vi "SCMP - Write FITS File v2 coop.vi"(6 "FITS Header":T1={"Wavelength (nm)"=530.15, "Exposure (s)"=0.05, "Tuning Delay (ms)"=1000.0, "Beam Type (-1/1)"=1.0, "Tuning Voltages"=[1.111, 2.222, 3.333, 4.444], "Observer"="observer", "Light Shapping Diffuser"=enum."In Beam", "Comment"="", "Data Type"=enum."HOLE", "Mod Cycles"=0, "SCD Calibration Optics"=enum."1 - Polarizer @0, I+Q", "SCD Emission Line Filter"=enum."1-557.6nm", "Cookbook"="", "COMP-S Calibration Wheel"=enum."Dark", "COMP-S Andover Filter Wheel"=enum."530.3nm/HWB 0.34nm (Fe XIV)", "FOV Rotation (deg)"=66.0, "Objective Lens Position (mm)"=0.0, "Occulter size"=0.0, "Time End"=timestamp(3382374145.421875 s since 1904-01-01), "Acc Exposure (s)"=0.0, "Time Stamp Array"=[], "Camera Serial Number"=[], "Camera Temp"=[], "Camera PI (mm)"=[], "Time Start"=timestamp(3382374145.421875 s since 1904-01-01), "Peripherals"={"ILX controler"=FALSE, "Zone temperatures"=FALSE, "Andor"=FALSE, "Andor 2"=FALSE, "PI Stages"=FALSE, "AISAS mechanisms"=FALSE, "AISAS Mech.lvclass"=refnum, "Zone temp ref"=variant, "FWs"=FALSE}, "FITS paths"=[], "Cameras"=enum."Andor", "load preset cbk"=FALSE, "periodic check count"=0, "COMP-S Calibration Wheel 2"=enum."Dark", "Calib"=enum."Dark", "Abso Aperture"=66.0, "Nominal Aperture"=66.0} {"Nominal Aperture" format="%.1f"; "Abso Aperture" format="%.1f"; "Camera PI (mm)" format="%_3g"; "Acc Exposure (s)" format="%^.3g"; "Occulter size" format="%.2f"; "Objective Lens Position (mm)" min=70.0 max=152.0 format="%.2f"; "FOV Rotation (deg)" format="%.1f"; "Exposure (s)" format="%^.3g"; "Wavelength (nm)" format="%_6g"}, 8 "error in":errorcluster, 9 "Image #":i32, 10 "Data":u32[][][](array[numeric]), 11 "Camera.lvclass":refnum<class "Camera.lvclass">) -> (0 "error out":errorcluster, 2 "FITS Path Out":path=path "G:/SCD Data/Level-0/20141030/20141030.160747.FTS")   [LabVIEW 2014]
doc: "Use this template to build a VI to use as a subVI."
uses:
  Controls/SCD - FITS Cluster.ctl
  AISAS/Mech/AISAS Mech.lvclass
  AISAS/Controls/Diffuser.ctl
  Controls/FITS Data type.ctl
  Controls/SCD - Calibration Optics Filter Wheel.ctl
  Controls/SCD - EDT - Emission Line Filter Wheel.ctl
  Controls/CoMP-S Controls/Polarization Optics Filter Wheel.ctl
  Controls/CoMP-S Controls/Emission Line Filter Wheel.ctl
  AISAS/Controls/focus.ctl
  Controls/peripherals.ctl
  Controls/Cameras select.ctl
  Camera/Camera/Camera.lvclass
panel:
  out "<ADU>":dbl[](array[numeric])
  in  "A":u32[][](array[numeric])
  in  "D":u32[][](array[numeric])
  in  "C":u32[][](array[numeric])
  in  "B":u32[][](array[numeric])
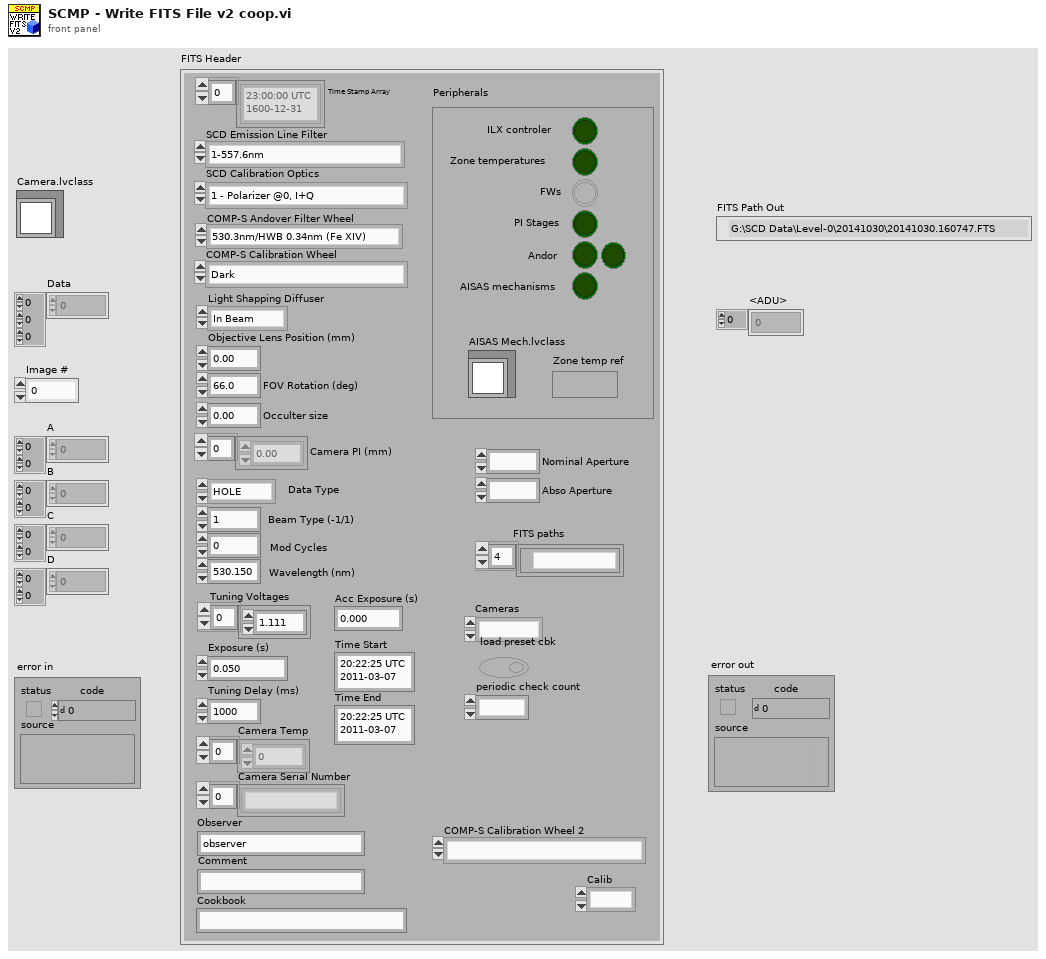
[diagram p1: front panel]
types:
  T1 = typedef "SCD - FITS Cluster.ctl" = cluster{"Wavelength (nm)":dbl, "Exposure (s)":dbl, "Tuning Delay (ms)":dbl, "Beam Type (-1/1)":dbl, "Tuning Voltages":dbl[], "Observer":string, "Light Shapping Diffuser":T2, "Comment":string, "Data Type":T3, "Mod Cycles":u16, "SCD Calibration Optics":T4, "SCD Emission Line Filter":T5, "Cookbook":string, "COMP-S Calibration Wheel":T6, "COMP-S Andover Filter Wheel":T7, "FOV Rotation (deg)":dbl, "Objective Lens Position (mm)":T8, "Occulter size":dbl, "Time End":timestamp, "Acc Exposure (s)":dbl, "Time Stamp Array":timestamp[], "Camera Serial Number":string[], "Camera Temp":dbl[], "Camera PI (mm)":dbl[], "Time Start":timestamp, "Peripherals":T9, "FITS paths":path[], "Cameras":T10, "load preset cbk":bool, "periodic check count":i32, "COMP-S Calibration Wheel 2":T6, "Calib":enum16{"Dark", "Flat"}, "Abso Aperture":dbl, "Nominal Aperture":dbl}
  T2 = typedef "Diffuser.ctl" = enum16{"Out of Beam", "In Beam"}
  T3 = typedef "FITS Data type.ctl" = enum16{"LIVE", "DARK", "FLAT", "CALI", "OBSE", "ABSO", "AURE", "TARG", "OBJE", "HOLE", "OREX", "THRO", "CHIP"}
  T4 = typedef "SCD - Calibration Optics Filter Wheel.ctl" = enum16{"1 - Polarizer @0, I+Q", "2 - Polarizer @90, I-Q", "3 - Polarizer @45, I+U", "4 - Polarizer @135, I-U", "5 - Polarizer @0, Retarder @45, I+V", "6 - Polarizer @0, Retarder @135, I-V", "7 - Dark", "8 - Clear", "9 - N/A"}
  T5 = typedef "SCD - EDT - Emission Line Filter Wheel.ctl" = enum16{"1-557.6nm", "2-587.6nm", "3-589.6nm", "4-630.2nm", "5-656.4nm", "6-849.8nm", "7-854.2nm", "8-866.2nm", "9-1083.0nm"}
  T6 = typedef "Polarization Optics Filter Wheel.ctl" = enum16{"Dark", "Clear", "Exchange Lens", "Polarizer @0, I+Q", "Polarizer @90, I-Q", "Polarizer @45, I+U", "Polarizer @135, I-U", "Polarizer @0, Retarder @45, I+V", "Polarizer @0, Retarder @135, I-V"}
  T7 = typedef "Emission Line Filter Wheel.ctl" = enum16{"530.3nm/HWB 0.34nm (Fe XIV)", "587.6nm/HBW 0.44nm (He I D3)", "637.5nm/HBW 0.53nm (Fe X)", "656.3nm/HBW 0.57nm (H-Alpha)", "789.2nm/HBW 0.85nm (Fe XI)", "854.2nm/HBW 1.01nm (Ca I)", "1074.7nm/HBW 2.34nm (Fe XIII)", "1079.8nm/HBW 1.64nm (Fe XIII)", "1083.0nm/HBW 1.66nm (He I)"}
  T8 = typedef "focus.ctl" = dbl
  T9 = typedef "peripherals.ctl" = cluster{"ILX controler":bool, "Zone temperatures":bool, "Andor":bool, "Andor 2":bool, "PI Stages":bool, "AISAS mechanisms":bool, "AISAS Mech.lvclass":refnum<class "AISAS Mech.lvclass">, "Zone temp ref":variant, "FWs":bool}
  T10 = typedef "Cameras select.ctl" = enum16{"Andor", "GDR"}
  T11 = typedef "beaning.ctl" = enum16{"1x1", "2x2", "3x3", "4x4", "8x8"}
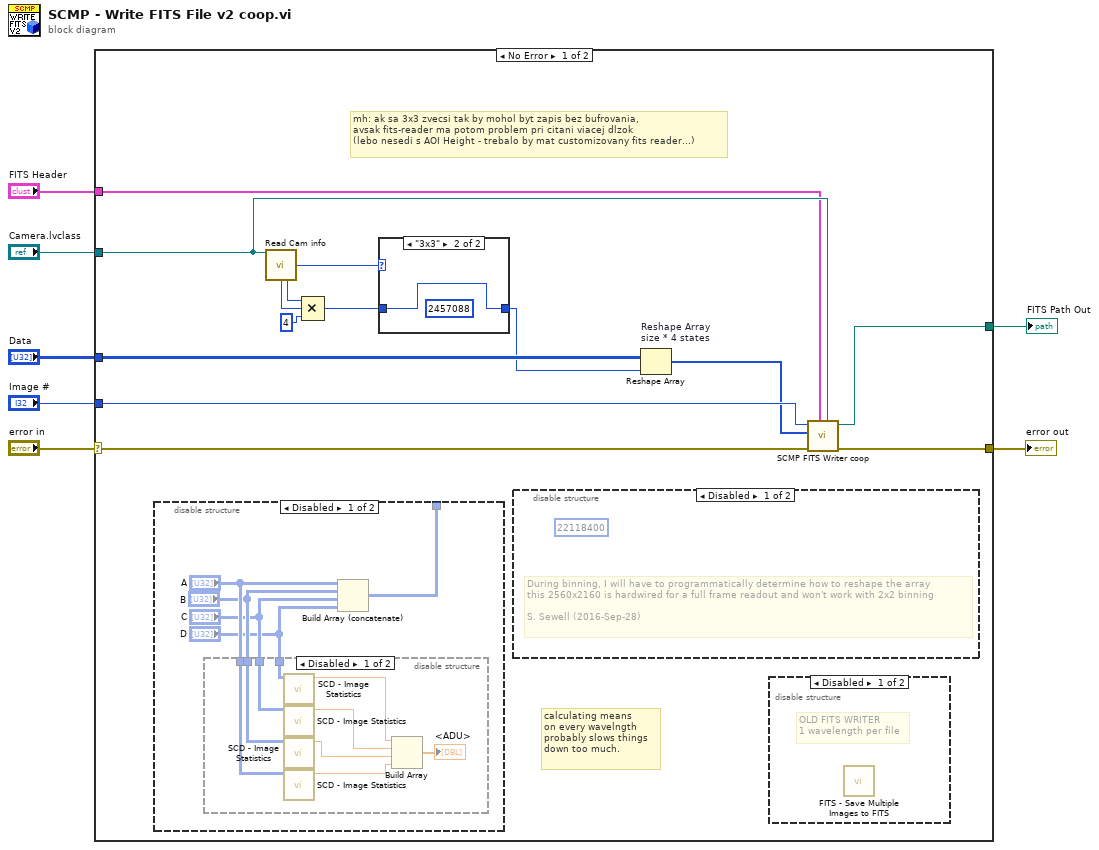
[diagram p0: block diagram]
diagram:
  n1 = case shown="No Error" "error in" {
    selector: "error in" -> [w8 w38]
    tunnel: [w21 w38] -> w7
    tunnel: "Camera.lvclass" -> [w20 _]
    tunnel: "FITS Header" -> [w19 _]
    tunnel: [w18 _] -> w4
    tunnel: "Data" -> [w17 _]
    tunnel: "Image #" -> [w16 _]
    frame No Error {
      # "calculating means\non every wavelngth\nprobably slows things\ndown too much."
      # "mh: ak sa 3x3 zvecsi tak by mohol byt zapis bez bufrovania, \navsak fits-reader ma potom problem pri citani viacej dlzok\n(lebo nesedi s AOI Height - trebalo by mat customizovany fits reader...)"
      n2 = disable-structure shown="Disabled" {
        disable-tunnel: [w28 _] -> _
        frame Disabled {
          n3 = disable-structure shown="Disabled" {
            disable-tunnel: "A" -> [w37 _]
            disable-tunnel: "B" -> [w36 _]
            disable-tunnel: "C" -> [w35 _]
            disable-tunnel: "D" -> [w34 _]
            frame Disabled {
              n4 = call "SCD - Image Statistics.vi"("I32 Image"=w34) -> ("mean"=w33:dbl)  [unwired: 9 in, 1 out]
              n5 = call "SCD - Image Statistics.vi"("I32 Image"=w35) -> ("mean"=w32:dbl)  [unwired: 9 in, 1 out]
              n6 = call "SCD - Image Statistics.vi"("I32 Image"=w36) -> ("mean"=w31:dbl)  [unwired: 9 in, 1 out]
              n7 = call "SCD - Image Statistics.vi"("I32 Image"=w37) -> ("mean"=w30:dbl)  [unwired: 9 in, 1 out]
              n8 = Build Array(w33, w32, w31, w30) -> (→"<ADU>":dbl[])
            }
            frame Enabled {
            }
          }
          n9 = Build Array (concatenate)("A", "B", "C", "D") -> (w28:u32[][])
        }
        frame Enabled {
        }
      }
      n10 = call-dynamic "Read Cam info.vi"("Camera in"=w20) -> ("Binning"=w10:T11, "AOI Width"=w11:i32, "AOI Height"=w12:i32)  [unwired: 5 in, 7 out]
      n11 = Compound Arithmetic op=MULTIPLY(w12, w11, 4 ("value")) -> (w14:i32)
      n12 = case shown="\"3x3\"" w10 {
        tunnel: w14 -> [w22 w23]
        tunnel: [w22 w23] -> w13
        frame "1x1", Default {
        }
        frame "3x3" {
          (unwired) 2457088 ("dimension size")
        }
      }
      n13 = disable-structure shown="Disabled" {
        frame Disabled {
          (unwired) 22118400 ("dimension size")
          # "During binning, I will have to programmatically determine how to reshape the array\nthis 2560x2160 is hardwired for a full frame readout and won't work with 2x2 binning\n\nS. Sewell (2016-Sep-28)"
        }
        frame Enabled {
        }
      }
      n14 = Reshape Array "Reshape Array\nsize * 4 states"(w17, w13) -> (w9:u32[])
      n15 = disable-structure shown="Disabled" {
        frame Disabled {
          # "OLD FITS WRITER\n1 wavelength per file"
          n16 = call "FITS - Save Multiple Images to FITS.vi"() -> ()  [unwired: 9 in, 3 out]
        }
        frame Enabled {
        }
      }
      n17 = call "SCMP FITS Writer coop.vi"("Camera.lvclass"=w20, "FITS Cluster"=w19, "error in"=w8, "Image Vector"=w9, "Wavelength (0..n)"=w16) -> ("error out"=w21:errorcluster, "Current FITS Path"=w18:path)  [unwired: 5 in]
    }
    frame Error {
    }
  }
  "error out" <- w7
  "FITS Path Out" <- w4
